vi "Find Pixel State.vi"(10 "V":i64, 11 "cycle":i64) -> (2 "Position":cluster{i64, i64}, 3 "State":bool)   [LabVIEW 2021, in "d10.lvlib"]
uses:
  d10.lvlib
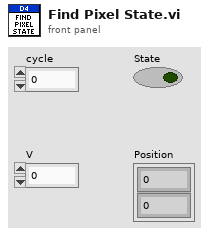
[diagram p1: front panel]
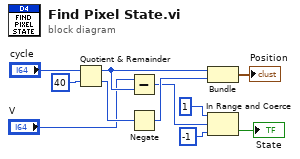
[diagram p0: block diagram]
diagram:
  n1 = Quotient & Remainder(x="cycle", y=i64 40) -> (x-y*floor(x/y)=w7:i64, floor(x/y)=w9:i64)
  n2 = Subtract(x="V", y=w7) -> (x-y=w2:i64)
  n3 = Negate(x=w9) -> (-x=w10:i64)
  n4 = Bundle(w7, w10) -> (→"Position":cluster{i64, i64})  [unwired: 1 in]
  n5 = In Range and Coerce(upper limit=i64 1, x=w2, lower limit=i64 -1) -> (In Range?=→"State":bool)  [unwired: 1 out]
